vi "Main4.vi"() -> ()   [LabVIEW 2014]
doc: "The myRIO Project template acquires acceleration data from the onboard accelerometer and displays the changes of acceleration values in a waveform chart."
uses:
  <vilib>/myRIO/Instrument Drivers/Onboard IO/AI/typedefs/AI Reference.ctl
  <vilib>/myRIO/Common/Instrument Driver Framework/Utilities/typedefs/myRIO Generic Hardware Reference.ctl
  <vilib>/myRIO/Common/Instrument Driver Framework/Utilities/typedefs/Hardware Version Enum.ctl
  <vilib>/myRIO/Common/Instrument Driver Framework/Utilities/typedefs/myRIO v1.0 Reference.ctl
  <vilib>/myRIO/Common/Instrument Driver Framework/Utilities/typedefs/Generic FPGA Reference.ctl
  <vilib>/myRIO/Common/Instrument Driver Framework/myRIO v1.0/AI/typedefs/AI Channels List.ctl
  <vilib>/myRIO/Common/Instrument Driver Framework/myRIO v1.0/AI/typedefs/AI Channels Enum.ctl
  <vilib>/myRIO/Common/Instrument Driver Framework/Utilities/typedefs/Analog Scaling Constants List.ctl
  <vilib>/myRIO/Common/Instrument Driver Framework/Utilities/typedefs/Analog Scaling Constants.ctl
  <vilib>/userdefined/High Color/nirio_resource_hc.ctl
  <vilib>/myRIO/Instrument Drivers/Onboard IO/PWM/typedefs/PWM Reference.ctl
  <vilib>/myRIO/Common/Instrument Driver Framework/myRIO v1.0/PWM/typedefs/PWM Channels Enum.ctl
  <vilib>/myRIO/Instrument Drivers/Onboard IO/PWM/typedefs/PWM Configuration.ctl
  <vilib>/myRIO/Instrument Drivers/Onboard IO/DIO/typedefs/DIO Reference.ctl
  <vilib>/myRIO/Common/Instrument Driver Framework/myRIO v1.0/DIO/typedefs/DIO Channels List.ctl
  <vilib>/myRIO/Common/Instrument Driver Framework/myRIO v1.0/DIO/typedefs/DIO Channels Enum.ctl
  <vilib>/myRIO/Common/Instrument Driver Framework/Utilities/vis/Is FPGA Ref Available.vi
  <vilib>/myRIO/Common/Instrument Driver Framework/myRIO v1.0/AI/vis/myRIO v1.1 Open AI.vi
  <vilib>/myRIO/Instrument Drivers/Onboard IO/AI/vis/Read.vi
  <vilib>/myRIO/Common/Instrument Driver Framework/myRIO v1.0/PWM/vis/myRIO v1.1 Open PWM.vi
  <vilib>/myRIO/Instrument Drivers/Onboard IO/PWM/vis/Set Duty Cycle and Frequency.vi
  <vilib>/myRIO/Common/Instrument Driver Framework/myRIO v1.0/DIO/vis/myRIO v1.1 Open DIO.vi
  <vilib>/myRIO/Instrument Drivers/Onboard IO/DIO/vis/Write.vi
  <vilib>/myRIO/Common/Instrument Driver Framework/Utilities/vis/Validate Channels.vi
  <vilib>/myRIO/Common/Instrument Driver Framework/myRIO v1.0/AI/vis/myRIO v1.0 Reserve AI.vi
  <vilib>/myRIO/Common/Instrument Driver Framework/myRIO v1.0/PWM/vis/myRIO v1.0 Reserve PWM.vi
  <vilib>/myRIO/Common/Instrument Driver Framework/myRIO v1.0/DIO/vis/myRIO v1.0 Reserve DIO.vi
  <vilib>/myRIO/Common/Instrument Driver Framework/myRIO v1.0/AI/vis/myRIO v1.0 Build MUX Configuration AI.vi
  <vilib>/myRIO/Common/Instrument Driver Framework/myRIO v1.0/Resource Manager/vis/myRIO v1.0 Reserve Channel List.vi
  <vilib>/myRIO/Common/Instrument Driver Framework/myRIO v1.0/PWM/vis/myRIO v1.0 Build MUX Configuration PWM.vi
  <vilib>/myRIO/Common/Instrument Driver Framework/myRIO v1.0/DIO/vis/myRIO v1.0 Build MUX Configuration DIO.vi
  <vilib>/myRIO/Common/Instrument Driver Framework/myRIO v1.0/Resource Manager/vis/myRIO v1.0 Reserve Channel.vi
  <vilib>/myRIO/Common/Instrument Driver Framework/myRIO v1.0/Resource Manager/vis/myRIO v1.0 Unreserve Channel.vi
  <vilib>/myRIO/Common/Instrument Driver Framework/myRIO v1.0/Resource Manager/vis/myRIO v1.0 Create Configuration List.vi
  <vilib>/myRIO/Common/Instrument Driver Framework/myRIO v1.0/Resource Manager/vis/myRIO v1.0 Build Mutex Name.vi
  <vilib>/Utility/VariantDataType/GetNumericInfo.vi
  <vilib>/Utility/error.llb/Error Cluster From Error Code.vi
  <vilib>/myRIO/Common/Instrument Driver Framework/myRIO v1.0/myRIO v1.1 Open.vi
  <vilib>/myRIO/Common/Instrument Driver Framework/myRIO v1.0/AI/vis/myRIO v1.0 Get Scaling Constants AI.vi
  <vilib>/myRIO/Common/Instrument Driver Framework/Utilities/vis/IO Manager.vi
  <vilib>/myRIO/Common/Instrument Driver Framework/Utilities/vis/Configuration Manager.vi
  <vilib>/myRIO/Common/Instrument Driver Framework/myRIO v1.0/myRIO v1.0 Close.vi
  <vilib>/myRIO/Common/Instrument Driver Framework/myRIO v1.0/AI/vis/myRIO v1.0 Read AI.vi
  <vilib>/myRIO/Common/Instrument Driver Framework/myRIO v1.0/Resource Manager/vis/myRIO v1.0 Configure IO.vi
  <vilib>/myRIO/Common/Instrument Driver Framework/myRIO v1.0/PWM/vis/myRIO v1.0 Write PWM.vi
  <vilib>/myRIO/Common/Instrument Driver Framework/myRIO v1.0/DIO/vis/myRIO v1.0 Write DIO.vi
  <vilib>/myRIO/Express VI/Onboard IO/AI/AI Express VI.xnode
  <vilib>/myRIO/Instrument Drivers/Onboard IO/AI/vis/myRIO AI Open.xnode
  <vilib>/myRIO/Express VI/Onboard IO/PWM/PWM Express VI.xnode
  <vilib>/myRIO/Instrument Drivers/Onboard IO/PWM/vis/myRIO PWM Open.xnode
  <vilib>/myRIO/Express VI/Onboard IO/DO/DO Express VI.xnode
  <vilib>/myRIO/Instrument Drivers/Onboard IO/DIO/vis/myRIO DIO Open.xnode
  <vilib>/myRIO/Instrument Drivers/Onboard IO/PWM/PWM.lvlib
  <vilib>/vision/driver/NI_Vision_Acquisition_Software.lvlib
  <vilib>/vision/NI_Vision_Development_Module.lvlib
  <vilib>/myRIO/Instrument Drivers/Onboard IO/AI/AI.lvlib
  <vilib>/myRIO/Instrument Drivers/Onboard IO/DIO/DIO.lvlib
panel:
  in  "x":bool
  in  "Number of Erosion":i32=4
  in  "Red or Hue":cluster{i32, i32}(slide)={0, 70} scale=0.0..255.0
  in  "Threshold Color Mode":enum32{"RGB", "HSL"}(radio)=enum."HSL"
  in  "Green or Saturation":cluster{i32, i32}(slide)={84, 244} scale=0.0..255.0
  in  "Blue or Luminance":cluster{i32, i32}(slide)={0, 255} scale=0.0..255.0
  out "웨이브폼 차트":dbl(graph)=0.019531252
  out "Image 2":T1(plugin-control)
  in  "Stop 2":bool
  out "Image":T1(plugin-control)
  in  "Camera Name":refnum<k21>="cam3" caption="IMAQdx Session"
  # "Control Motor"
  # "Read Encoder"
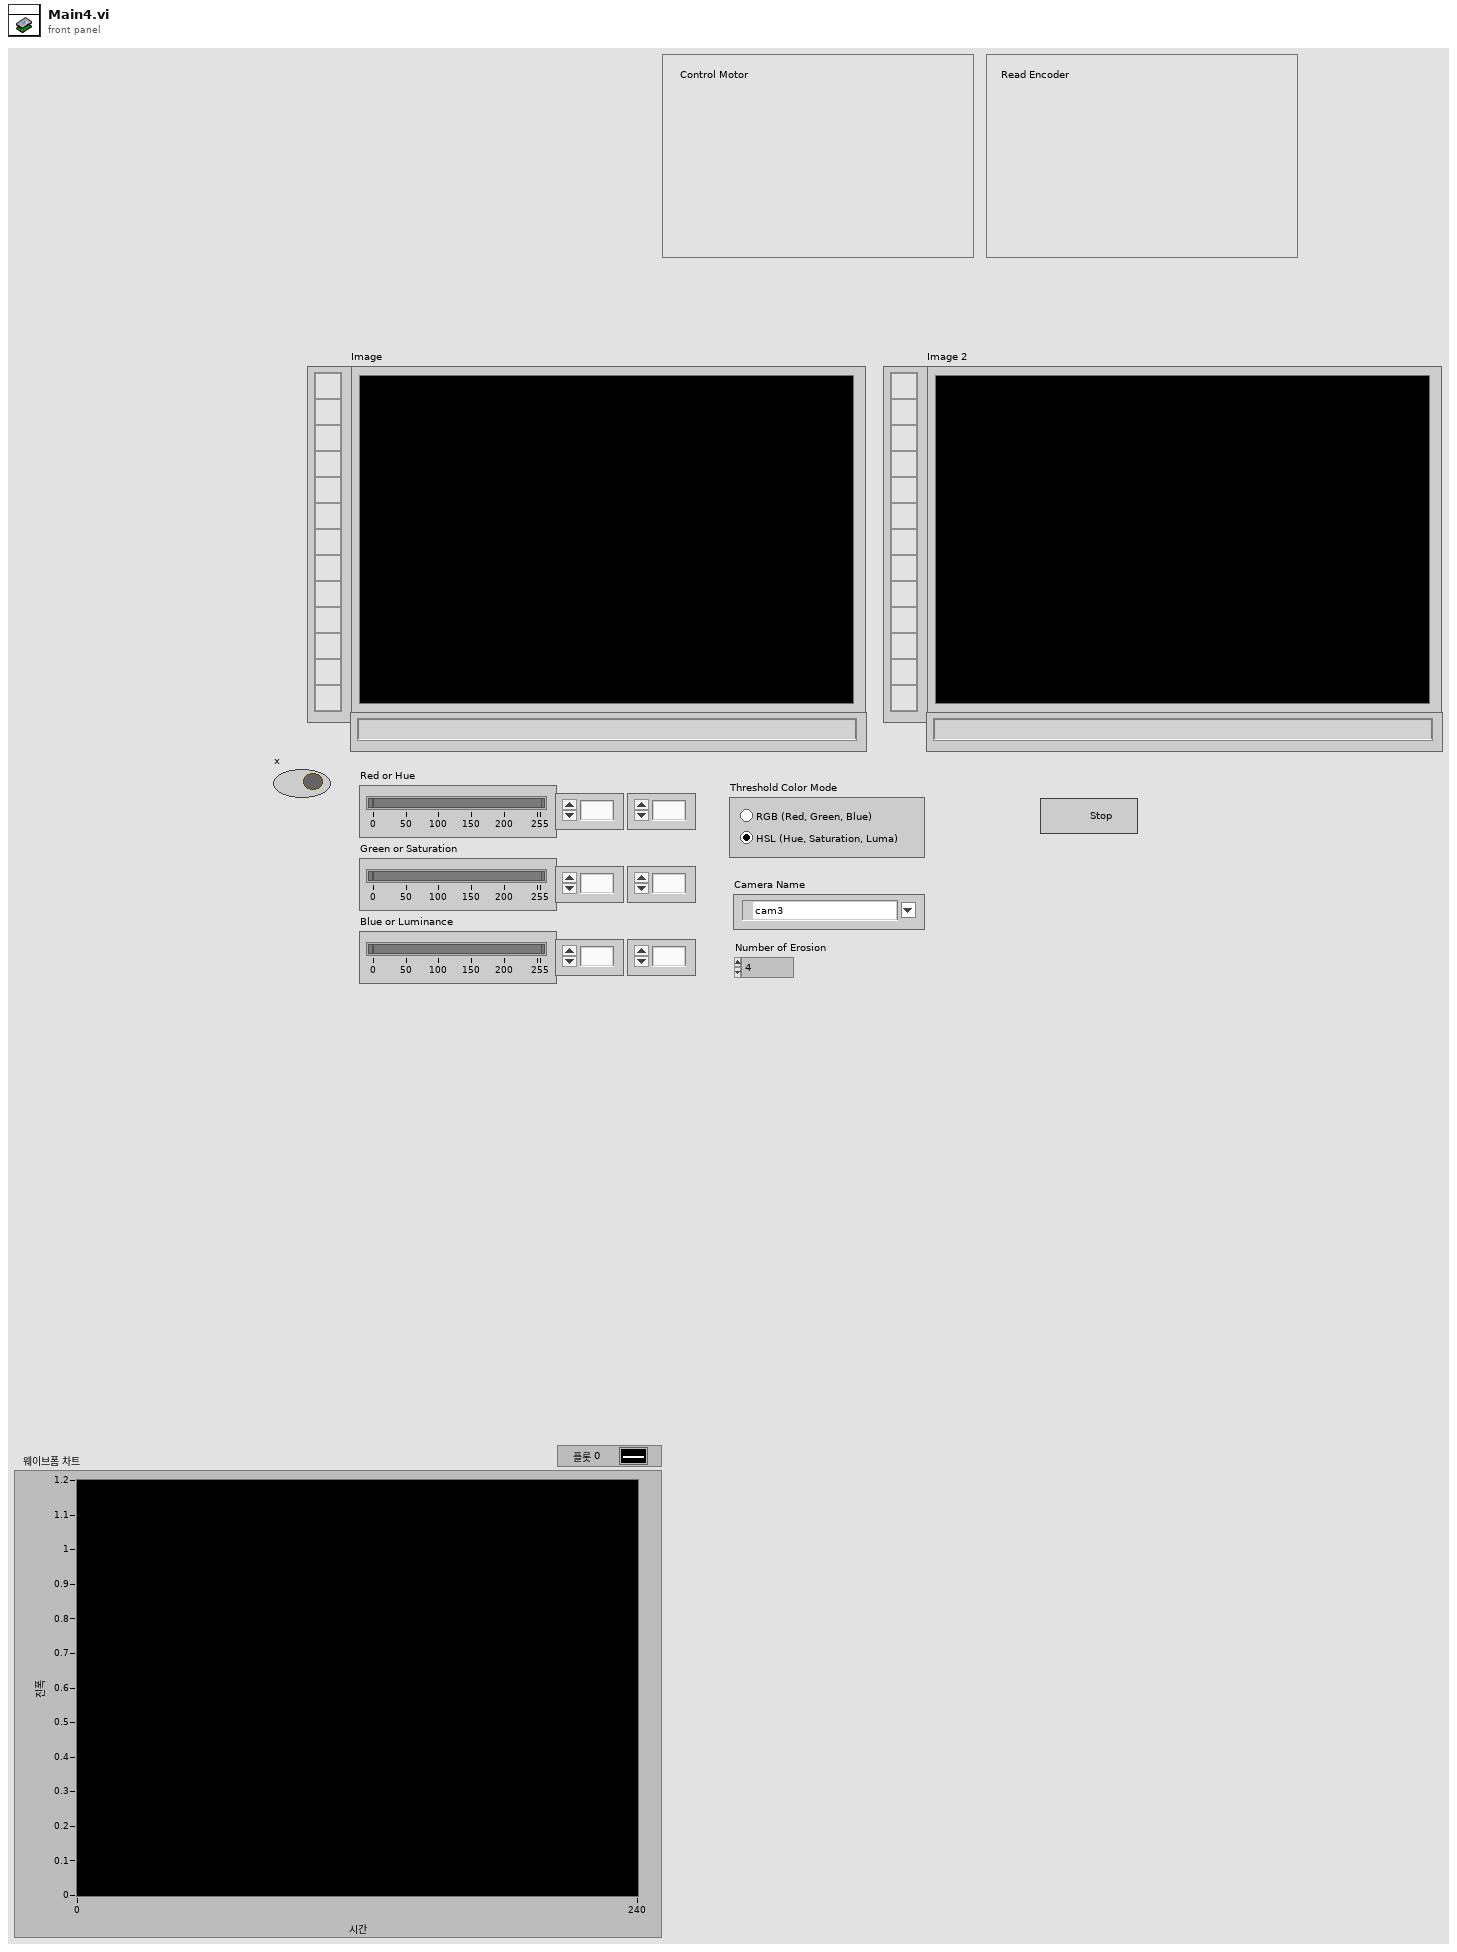
[diagram p1: front panel]
types:
  T1 = typedef "IMAQ Image.ctl" = refnum<image>
  T2 = typedef "DIO.lvlib/DIO Reference.ctl" = cluster{"myRIO Reference":T3, "DIO Channels List":T7}
  T3 = typedef "myRIO Generic Hardware Reference.ctl" = cluster{"myRIO Model":T4, "myRIO Hardware Reference":T5}
  T4 = typedef "Hardware Version Enum.ctl" = enum16{"Unknown", "myRIO-1900", "myRIO-1950"}
  T5 = typedef "myRIO v1.0 Reference.ctl" = cluster{"Generic FPGA Reference":T6, "Allow multiple opens":bool}
  T6 = typedef "Generic FPGA Reference.ctl" = refnum<k20>
  T7 = typedef "DIO Channels List.ctl" = T8[]
  T8 = typedef "DIO Channels Enum.ctl" = enum16{"Not Connected", "C/DIO0", "C/DIO1", "C/DIO2", "C/DIO3", "C/DIO4", "C/DIO5", "C/DIO6", "C/DIO7", "A/DIO0", "A/DIO1", "A/DIO2", "A/DIO3", "A/DIO4", "A/DIO5", "A/DIO6", "A/DIO7", "A/DIO8", "A/DIO9", "A/DIO10", "A/DIO11", "A/DIO12", "A/DIO13", "A/DIO14", "A/DIO15", "B/DIO0", "B/DIO1", "B/DIO2", "B/DIO3", "B/DIO4", "B/DIO5", "B/DIO6", "B/DIO7", "B/DIO8", "B/DIO9", "B/DIO10", "B/DIO11", "B/DIO12", "B/DIO13", "B/DIO14", "B/DIO15", "LED0", "LED1", "LED2", "LED3", "Button0"}
  T9 = typedef "nirio_resource_hc.ctl" = tag
  T10 = typedef "AI.lvlib/AI Reference.ctl" = cluster{"myRIO Reference":T3, "AI Channels List":T11, "AI Scaling Constants List":T13}
  T11 = typedef "AI Channels List.ctl" = T12[]
  T12 = typedef "AI Channels Enum.ctl" = enum16{"Not Connected", "AudioIn/Left", "AudioIn/Right", "C/AI0", "C/AI1", "A/AI0", "A/AI1", "A/AI2", "A/AI3", "B/AI0", "B/AI1", "B/AI2", "B/AI3"}
  T13 = typedef "Analog Scaling Constants List.ctl" = T14[]
  T14 = typedef "Analog Scaling Constants.ctl" = cluster{"LSB Weight (Volts)":dbl, "Offset (Volts)":dbl, "Signed?":bool}
  T15 = typedef "IMAQ Rectangle" = cluster{"Left":i32, "Top":i32, "Right":i32, "Bottom":i32, "Rotation":dbl}
  T16 = typedef "PWM.lvlib/PWM Reference.ctl" = cluster{"myRIO Reference":T3, "PWM Channels Enum":T17, "PWM Configuration":T18}
  T17 = typedef "PWM Channels Enum.ctl" = enum16{"Not Connected", "C/PWM0", "C/PWM1", "A/PWM0", "A/PWM1", "A/PWM2", "B/PWM0", "B/PWM1", "B/PWM2"}
  T18 = typedef "PWM.lvlib/PWM Configuration.ctl" = cluster{"Frequency":dbl, "Duty Cycle":dbl}
  T19 = typedef "Image Type" = u32
  T20 = typedef "IMAQdx.ctl" = refnum<k21>
  T21 = cluster{"Global Rectangle":i32[], "Contours":cluster{"Contour Type":u32, "ROI Type":u32, "Points":i32[]}[]}
  T22 = cluster{"Area":dbl, "Number of Holes":dbl, "Bounding Rect":cluster{"Left":dbl, "Top":dbl, "Right":dbl, "Bottom":dbl}, "Center of Mass":cluster{"X":dbl, "Y":dbl}, "Orientation":dbl, "Dimensions":cluster{"Width":dbl, "Height":dbl}}[]
  T23 = cluster{"Left":dbl, "Top":dbl, "Right":dbl, "Bottom":dbl}
  T24 = typedef "ROI Descriptor" = cluster{"Global Rectangle":i32[], "Contours":cluster{"ID":enum32{"External", "Internal"}, "Type":u32, "Coordinates":i32[]}[]}
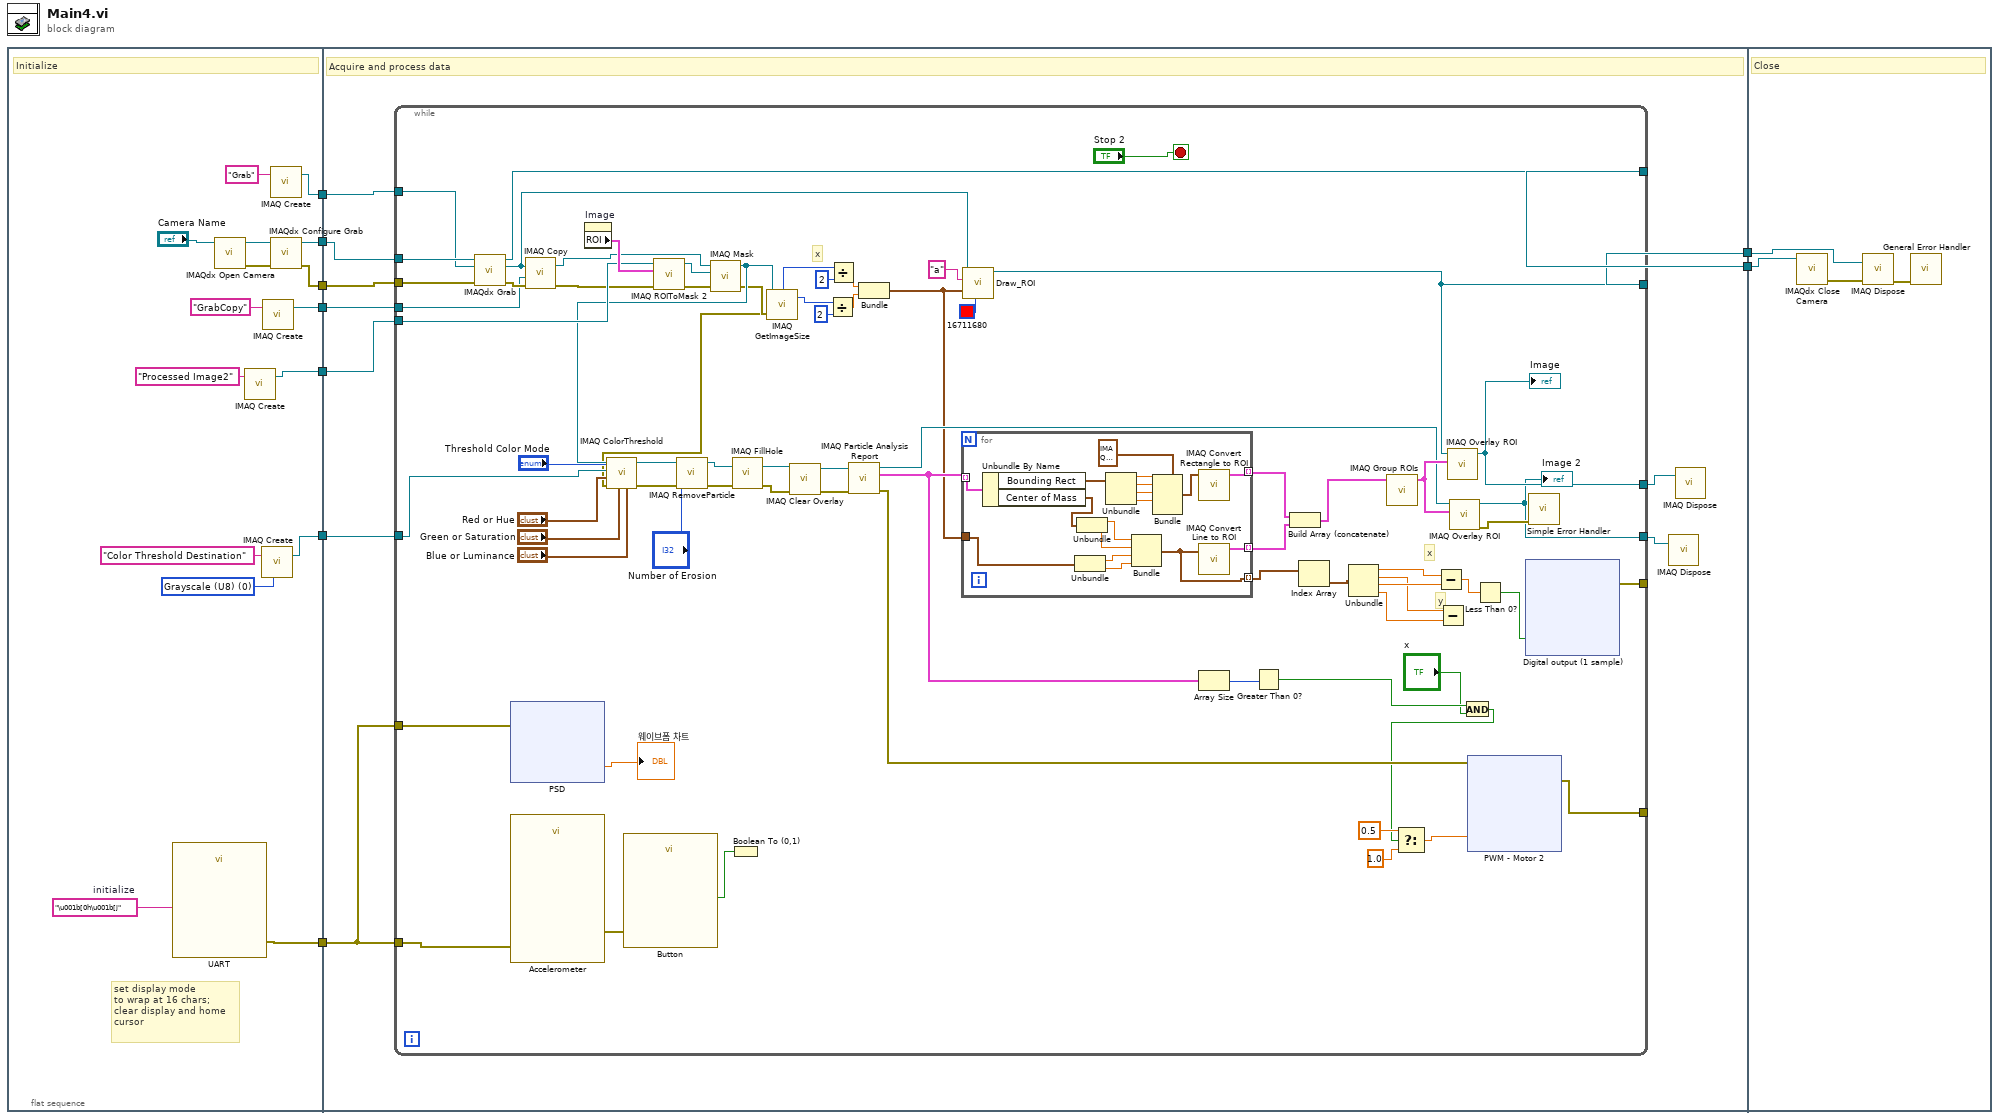
[diagram p0: block diagram]
diagram:
  n1 = flat-sequence {
    tunnel: [w21] -> w9
    tunnel: [w20] -> w8
    tunnel: [w19] -> w7
    tunnel: [w17] -> w4
    tunnel: [w15] -> w3
    tunnel: [w14] -> w2
    tunnel: [w10] -> w1
    tunnel: w9 -> [w36]
    tunnel: w8 -> [w35]
    tunnel: w7 -> [w34]
    tunnel: [w28] -> w6
    tunnel: [w33] -> w5
    tunnel: w4 -> [w30]
    tunnel: w3 -> [w29]
    tunnel: w2 -> [w27]
    tunnel: w1 -> [w26]
    tunnel: w6 -> [w235]
    tunnel: w5 -> [w234]
    frame #0 {
      w12 = T19 0 items=["Grayscale (U8)", "Grayscale (I16)", "Grayscale (SGL)", "Complex (CSG)", "RGB (U32)", "HSL (U32)", "RGB (U64)", "Grayscale (U16)"] ("Image Type")
      w13 = "\u001b[0h\u001b[j"  # initialize
      # "set display mode\nto wrap at 16 chars;\nclear display and home\ncursor"
      # "Initialize"
      n2 = call "UART"("Characters to Write"=w13) -> ("error out"=w14:errorcluster)  [unwired: 25 in, 1 out]
      n3 = call <vilib>:"IMAQdx Open Camera.vi"("Session In"="Camera Name") -> ("error out"=w25:errorcluster, "Session Out"=w24:T20)  [unwired: 2 in, 7 out]
      n4 = call "IMAQ Create"("Image Name"="Processed Image2") -> ("New Image"=w17:T1)  [unwired: 3 in, 2 out]
      n5 = call "IMAQ Create"("Image Name"="Color Threshold Destination", "Image Type"=w12) -> ("New Image"=w10:T1)  [unwired: 3 in, 1 out]
      n6 = call "IMAQ Create"("Image Name"="GrabCopy") -> ("New Image"=w15:T1)  [unwired: 3 in, 2 out]
      n7 = call "IMAQ Create"("Image Name"="Grab") -> ("New Image"=w21:T1)  [unwired: 3 in, 2 out]
      n8 = call <vilib>:"IMAQdx Configure Grab.vi"("error in"=w25, "Session In"=w24) -> ("error out"=w19:errorcluster, "Session Out"=w20:T20)  [unwired: 8 out]
    }
    frame #1 {
      # "Acquire and process data"
      n9 = while {
        tunnel: [w106] -> w33
        tunnel: w34 -> [w108]
        tunnel: w35 -> [w109]
        tunnel: w36 -> [w107]
        tunnel: [w103] -> _
        tunnel: [w70] -> w32
        tunnel: [w69] -> w31
        tunnel: w30 -> [w93]
        tunnel: w29 -> [w78]
        tunnel: [w71] -> w28
        tunnel: w27 -> [w65]
        tunnel: w27 -> [w56]
        tunnel: w26 -> [w55]
        tunnel: [w37] -> _
        stop <- "Stop 2" stop-if-true
        # "y"
        # "x"
        # "x"
        n10 = call <vilib>:"IMAQdx Grab.vi"("error in"=w108, "Image In"=w107, "Session In"=w109) -> ("error out"=w80:errorcluster, "Image Out"=w76:T1, "Session Out"=w106:T20)  [unwired: 1 in, 5 out]
        n11 = xnode "PSD"("error in (no error)"=w56) -> ("C/AI0 (C/AI0 (AI0))"=→"웨이브폼 차트":dbl)  [unwired: 1 out]
        n12 = call "Accelerometer"("error in (no error)"=w65) -> ("error out"=w66:errorcluster)  [unwired: 23 in, 3 out]
        n13 = call "IMAQ Copy"("error in (no error)"=w80, "Image Dst"=w78, "Image Src"=w76) -> ("error out"=w79:errorcluster, "Image Dst Out"=w77:T1)  [unwired: 3 in]
        n14 = property on="Image" class="ImageControl"() -> ("ROI"=w95:T21)  [unwired: 2 in, 2 out]
        n15 = call "Button"("error in (no error)"=w66) -> ("Value"=w67:bool)  [unwired: 25 in, 1 out]
        n16 = call "IMAQ ROIToMask 2"("error in (no error)"=w79, "ROI Descriptor"=w95, "Image"=w93) -> ("error out"=w91:errorcluster, "Image Out"=w92:T1)  [unwired: 6 in, 1 out]
        n17 = call "IMAQ Mask"("error in (no error)"=w91, "Image Mask"=w92, "Image Src"=w77) -> ("error out"=w68:errorcluster, "Image Dst Out"=w75:T1)  [unwired: 2 in]
        n18 = Boolean To (0,1)(Boolean=w67) -> ()  [unwired: 1 out]
        n19 = call "IMAQ GetImageSize"("Image"=w75, "error in (no error)"=w68) -> ("Y Resolution"=w85:i32, "X Resolution"=w88:i32, "error out"=w47:errorcluster)  [unwired: 2 in]
        n20 = call "IMAQ ColorThreshold"("Blue or Luma or Val or Inten Range"="Blue or Luminance", "Green or Sat Range"="Green or Saturation", "Color Mode"="Threshold Color Mode", "error in (no error)"=w47, "Red or Hue Range"="Red or Hue", "Image Dst"=w55, "Image Src"=w75) -> ("error out"=w48:errorcluster, "Image Dst Out"=w50:T1)  [unwired: 3 in]
        n21 = call "IMAQ RemoveParticle"("error in (no error)"=w48, "Number of Erosion"="Number of Erosion", "Image Src"=w50) -> ("error out"=w43:errorcluster, "Image Dst Out"=w44:T1)  [unwired: 7 in]
        n22 = call "IMAQ FillHole"("error in (no error)"=w43, "Image Src"=w44) -> ("error out"=w46:errorcluster, "Image Dst Out"=w45:T1)  [unwired: 4 in]
        n23 = call "IMAQ Clear Overlay"("error in (no error)"=w46, "Image"=w45) -> ("error out"=w89:errorcluster, "Image Out"=w98:T1)  [unwired: 1 in, 7 out]
        n24 = Divide(x=w85, y=2) -> (x/y=w83:dbl)
        n25 = Divide(x=w88, y=2) -> (x/y=w84:dbl)
        n26 = call "IMAQ Particle Analysis Report"("error in (no error)"=w89, "Image"=w98) -> ("error out"=w96:errorcluster, "Particle Reports (Pixels)"=w90:T22, "Image Out (duplicate)"=w97:T1)  [unwired: 4 in, 3 out]
        n27 = Bundle(w84, w83) -> (w74:cluster{dbl, dbl})  [unwired: 1 in]
        n28 = for {
          tunnel: w90 -> [w198] mode=indexing
          tunnel: [w190] -> w73 mode=indexing
          tunnel: w74 -> [w186]
          tunnel: [w183] -> w64 mode=indexing
          tunnel: [w182] -> w63 mode=indexing
          n29 = Unbundle By Name(w198) -> ("Bounding Rect"=w196:T23, "Center of Mass"=w189:cluster{"X":dbl, "Y":dbl})
          n30 = Unbundle(w186) -> (w185:dbl, w184:dbl)
          n31 = Unbundle(w189) -> ("X"=w188:dbl, "Y"=w187:dbl)
          n32 = Unbundle(w196) -> ("Left"=w195:dbl, "Top"=w194:dbl, "Right"=w193:dbl, "Bottom"=w192:dbl)
          n33 = Bundle("X"=w188, "Y"=w187, w185, w184) -> (w182:cluster{"X":dbl, "Y":dbl, dbl, dbl})  [unwired: 1 in]
          n34 = Bundle(cluster=T15 {"Left"=0, "Top"=0, "Right"=0, "Bottom"=0, "Rotation"=0.0} ("Rectangle"), "Left"=w195, "Top"=w194, "Right"=w193, "Bottom"=w192) -> (w191:T15)  [unwired: 1 in]
          n35 = call "IMAQ Convert Rectangle to ROI"("Rectangle"=w191) -> ("ROI Descriptor"=w190:T24)  [unwired: 8 in, 1 out]
          n36 = call "IMAQ Convert Line to ROI"("Line"=w182) -> ("ROI Descriptor"=w183:T24)  [unwired: 8 in, 1 out]
        }
        n37 = call "Draw_ROI.vi"("Color"=u32 16711680, "클러스터"=w74, "Group"="a", "참조 번호 입력"=w76) -> ("참조 번호 출력"=w71:T1)  [unwired: 7 in]
        n38 = Array Size(array=w90) -> (size(s)=w102:i32)
        n39 = Greater Than 0?(x=w102) -> (x > 0?=w42:bool)
        n40 = Build Array (concatenate)(w73, w64) -> (w72:T24[])
        n41 = Index Array(array=w63) -> (element=w62:cluster{"X":dbl, "Y":dbl, dbl, dbl})  [unwired: 1 in]
        n42 = Unbundle(w62) -> ("X"=w61:dbl, "Y"=w59:dbl, w60:dbl, w58:dbl)
        n43 = call "IMAQ Group ROIs"("ROI Descriptors"=w72) -> ("ROI Descriptor out"=w104:T24)  [unwired: 1 in, 3 out]
        n44 = Subtract(x=w61, y=w60) -> (x-y=w39:dbl)
        n45 = Subtract(x=w59, y=w58) -> ()  [unwired: 1 out]
        n46 = call "IMAQ Overlay ROI"("ROI Descriptor"=w104, "Image"=w71) -> ("Image Out"=w70:T1)  [unwired: 4 in, 5 out]
        "Image" <- w70
        n47 = call "IMAQ Overlay ROI"("ROI Descriptor"=w104, "Image"=w97) -> ("error out"=w105:errorcluster, "Image Out"=w69:T1)  [unwired: 4 in, 4 out]
        "Image 2" <- w69
        n48 = And(x=w42, y="x") -> (x .and. y?=w41:bool)
        n49 = Select(t=0.5, s=w41, f=1.0) -> (s? t:f=w99:dbl)
        n50 = xnode "PWM - Motor 2"("Duty Cycle"=w99, "error in (no error)"=w96) -> ("error out"=w103:errorcluster)
        n51 = Less Than 0?(x=w39) -> (x < 0?=w38:bool)
        n52 = xnode "Digital output (1 sample)"("DIR0 (A/DIO6 (Pin 23))"=w38) -> ("error out"=w37:errorcluster)  [unwired: 1 in]
        n53 = call <vilib>:"Simple Error Handler.vi"("error in (no error)"=w105) -> ()  [unwired: 1 in, 8 out]
      }
      n54 = call "IMAQ Dispose"("Image"=w31) -> ()  [unwired: 5 in, 1 out]
      n55 = call "IMAQ Dispose"("Image"=w32) -> ()  [unwired: 5 in, 1 out]
    }
    frame #2 {
      # "Close"
      n56 = call <vilib>:"IMAQdx Close Camera.vi"("Session In"=w234) -> ("error out"=w237:errorcluster)  [unwired: 1 in, 9 out]
      n57 = call "IMAQ Dispose"("Image"=w235, "error in (no error)"=w237) -> ("error out"=w236:errorcluster)  [unwired: 4 in]
      n58 = call <vilib>:"General Error Handler.vi"("error in (no error)"=w236) -> ()  [unwired: 2 in, 13 out]
    }
  }
